vi "JSON Delta DIO Update.vi"(9 "Delta JSON":string, 11 "input":T1={"type"="DIO", "device"="", "name"="", "data"={"<init"=FALSE, "<>value"=FALSE, "<pulse_length"=0, "<input"=FALSE}}) -> (0 "error out":errorcluster, 3 "ouotput":T1={"type"="DIO", "device"="", "name"="", "data"={"<init"=FALSE, "<>value"=FALSE, "<pulse_length"=0, "<input"=FALSE}})   [LabVIEW 2019]
uses:
  DIO data proto.ctl
  DIO proto.ctl
panel:
  out "JSON of original":string
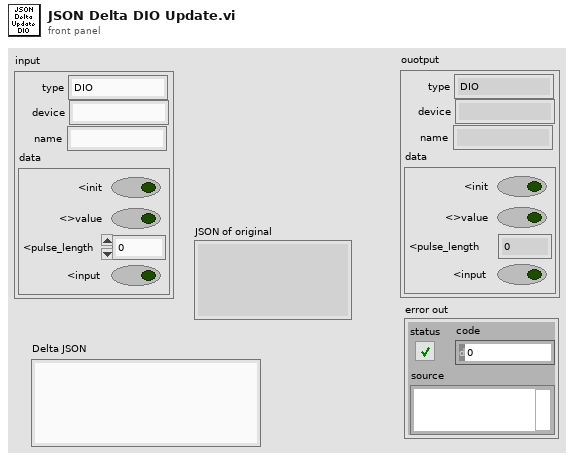
[diagram p1: front panel]
types:
  T1 = typedef "DIO proto.ctl" = cluster{"type":string, "device":string, "name":string, "data":T2}
  T2 = typedef "DIO data proto.ctl" = cluster{"<init":bool, "<>value":bool, "<pulse_length":i32, "<input":bool}
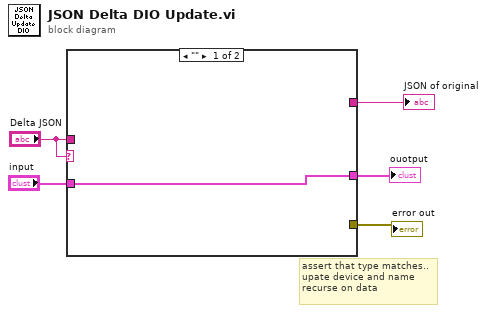
[diagram p0: block diagram]
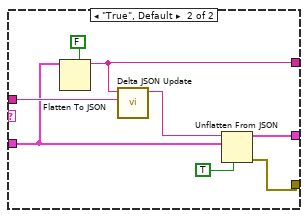
[diagram p2: hidden frame]
diagram:
  # "assert that type matches..\nupate device and name\nrecurse on data"
  n1 = case shown="\"\"" "Delta JSON" {
    tunnel: [_ w13] -> w5
    tunnel: "Delta JSON" -> [_ w11]
    tunnel: [_ w10] -> w4
    tunnel: "input" -> [w6 w8]
    tunnel: [w6 w7] -> w2
    frame "" {
    }
    frame "True", Default {
      n2 = Flatten To JSON(enable LabVIEW extensions? (T)=FALSE, anything=w8) -> (JSON string=w13:string)  [unwired: 1 in, 1 out]
      n3 = call "Delta JSON Update.vi"("Delta JSON"=w11, "JSON string in"=w13) -> ("JSON string out"=w12:string)  [unwired: 9 in]
      n4 = Unflatten From JSON(JSON string=w12, type and defaults=w8, default null elements? (F)=TRUE) -> (value=w7:T1, error out=w10:errorcluster)  [unwired: 4 in]
    }
  }
  "JSON of original" <- w5
  "error out" <- w4
  "ouotput" <- w2
